vi "The Plant and its parameters (v. 2021).vi"() -> ()   [LabVIEW 2021]
uses:
  <vilib>/addons/control/pid/pid.llb/PID Advanced (DBL).vi
  <vilib>/addons/control/pid/NI_PID_pid.lvlib
panel:
  out "Chart 2":dbl(graph)
  out "u-1":dbl
  out "u":dbl
  out "tank level":dbl
  out "Plant Output":dbl(slide) scale=0.0..100.0
  out "Error test":bool
  out "value":bool
  out "control signal variation":T1(graph)
  out "?":dbl[][](array[numeric])
  in  "set point":dbl=85.0
  in  "PID parameter":cluster{"K":dbl, "Ti (min)":dbl, "Td (min)":dbl}={"K"=5.0, "Ti (min)"=0.005, "Td (min)"=0.0}
  in  "Plant Parameters":T2={"Static Gain"=1.0, "lag (s)"=5.0, "deadtime (s)"=0.2, "load"=20.0, "deadband"=0.0, "sensor noise"=0.0, "initial PV"=0.0, "plant noise"=10.0}
  in  "?":bool
  # "output value"
  # "time"
  # "error"
  # "Leakage"
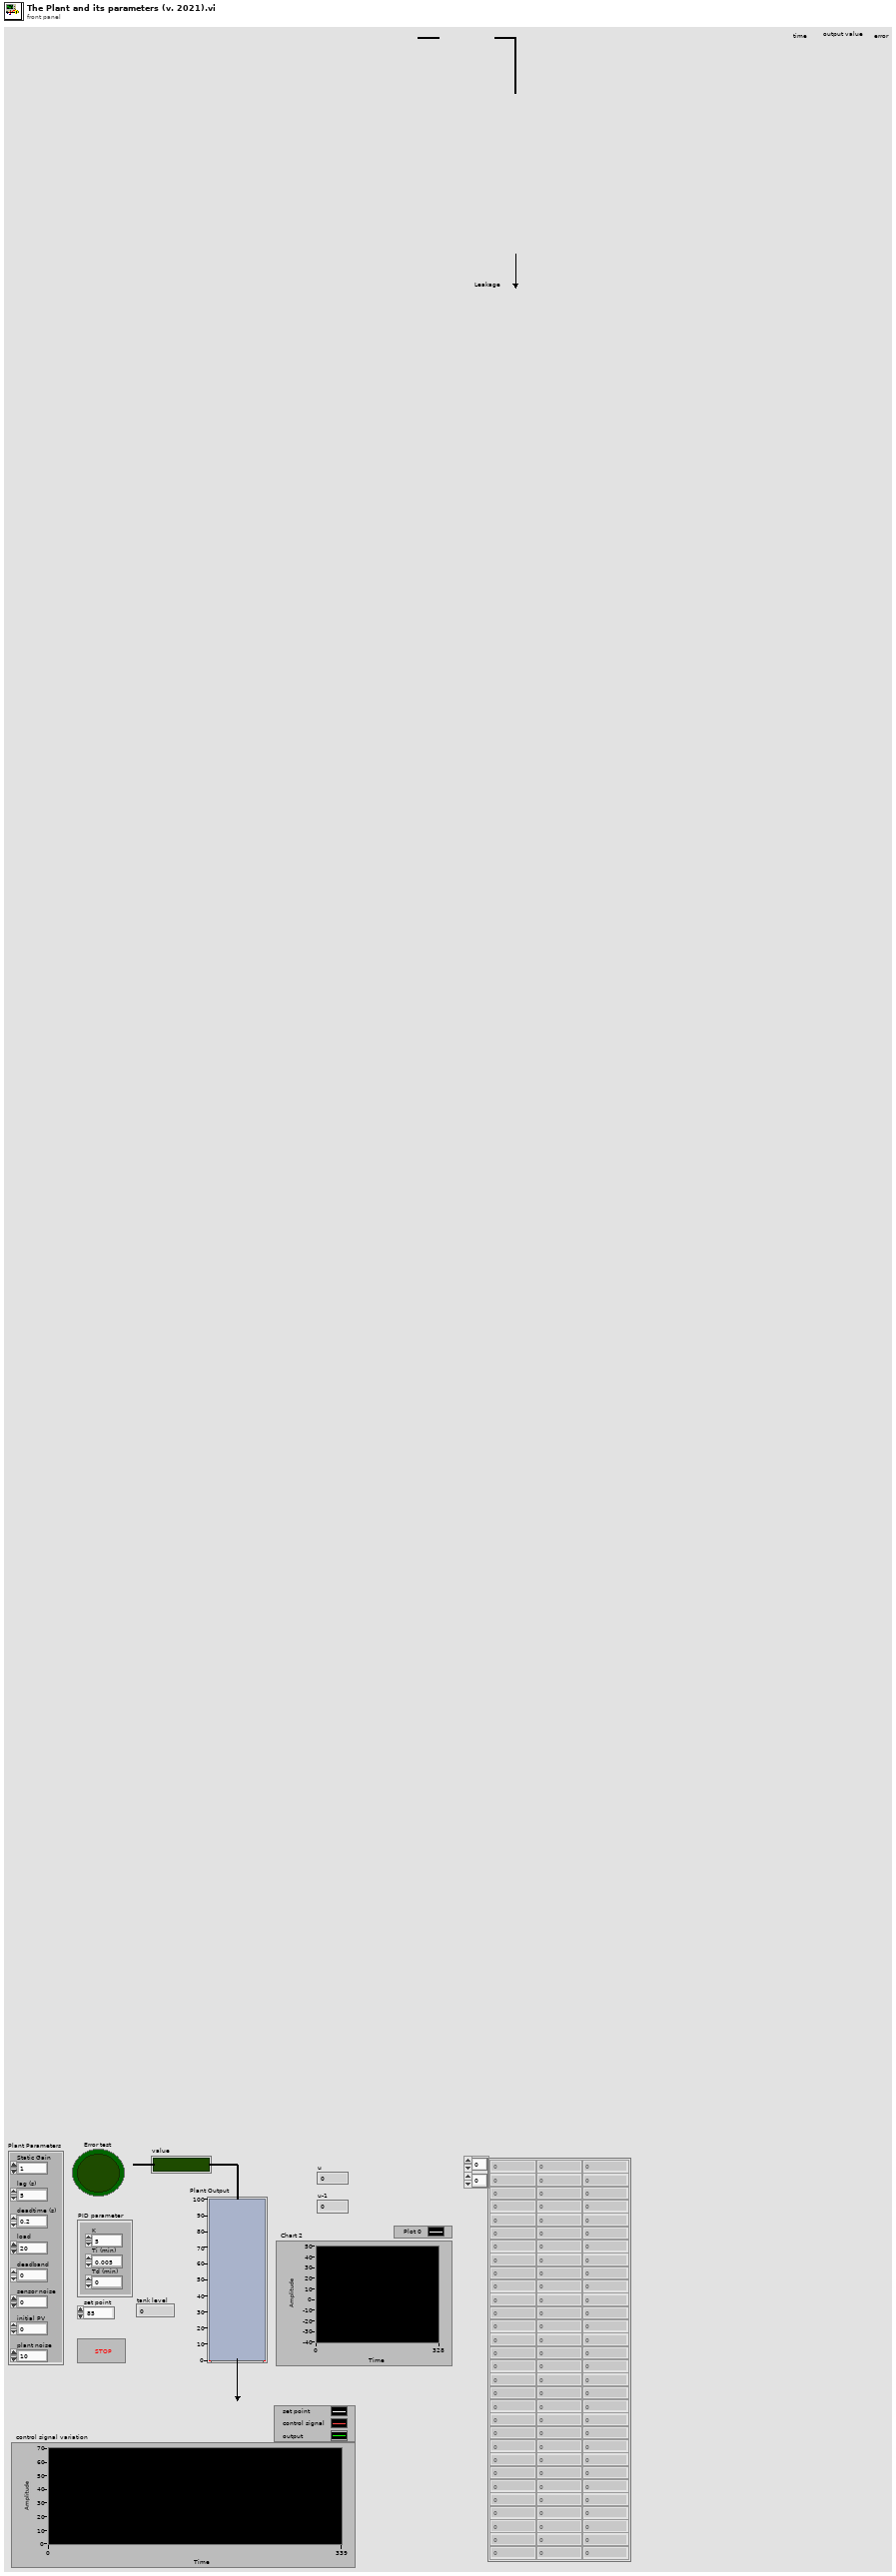
[diagram p1: front panel]
types:
  T1 = cluster{"set point":dbl, "output":dbl, "Plant Output":dbl}
  T2 = cluster{"Static Gain":dbl, "lag (s)":dbl, "deadtime (s)":dbl, "load":dbl, "deadband":dbl, "sensor noise":dbl, "initial PV":dbl, "plant noise":dbl}
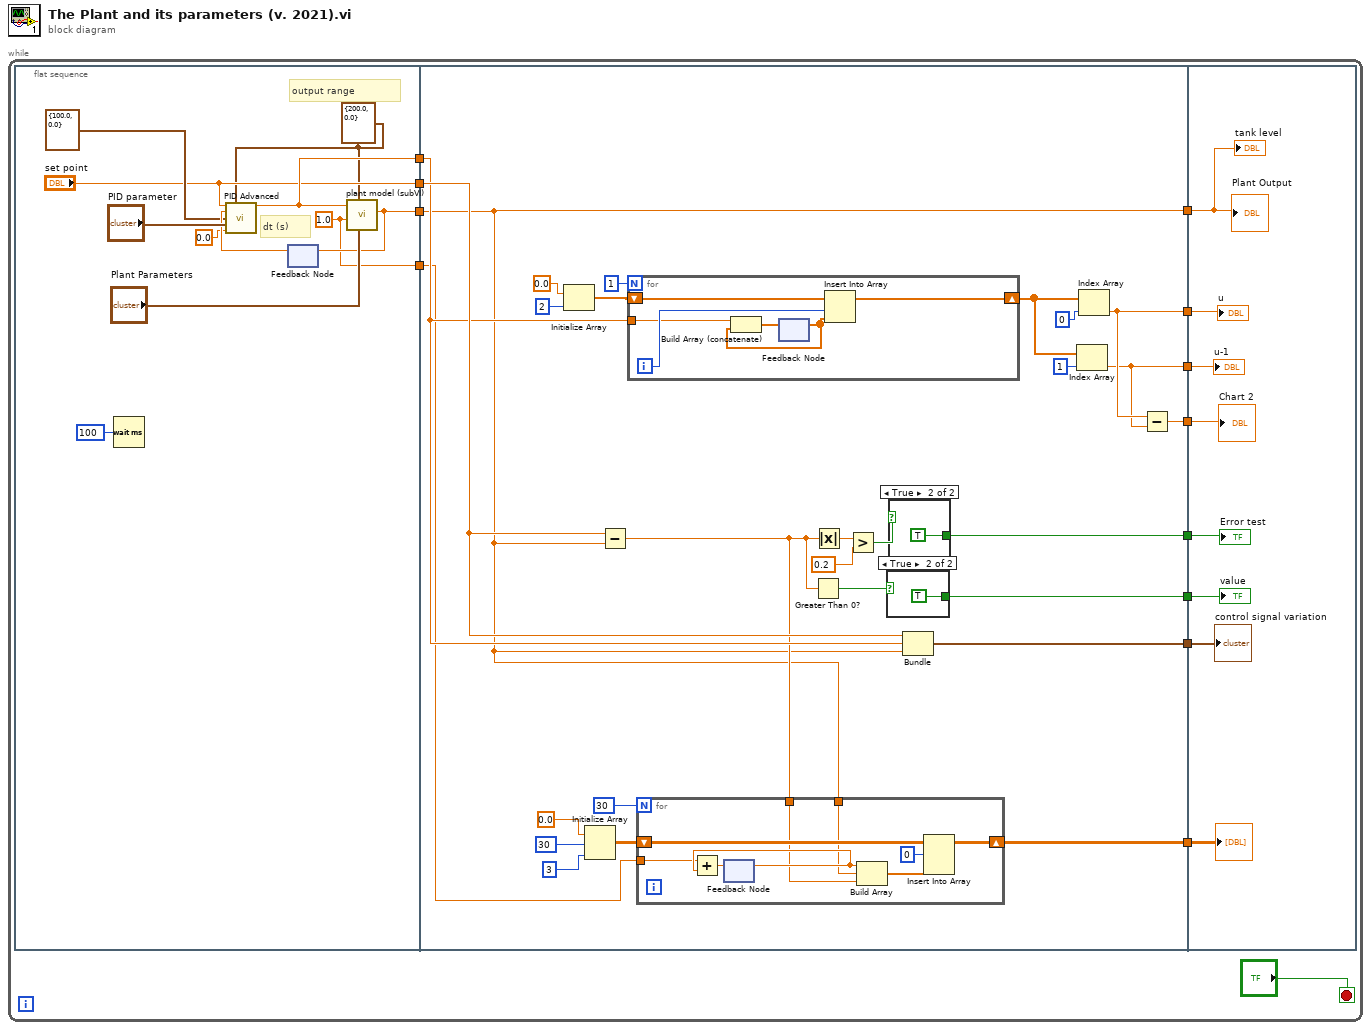
[diagram p0: block diagram]
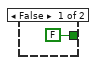
[diagram p2: hidden frame]
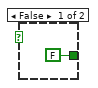
[diagram p3: hidden frame]
diagram:
  n1 = while {
    stop <- "?" stop-if-true
    n2 = flat-sequence {
      tunnel: [w19] -> w12
      tunnel: [w18] -> w11
      tunnel: ["set point"] -> w10
      tunnel: [w16] -> w1
      tunnel: w12 -> [w25]
      tunnel: w11 -> [w35]
      tunnel: w10 -> [w36]
      tunnel: [w34] -> w9
      tunnel: [w33] -> w8
      tunnel: [w32] -> w7
      tunnel: [w30] -> w6
      tunnel: [w29] -> w5
      tunnel: [w28] -> w4
      tunnel: [w27] -> w3
      tunnel: [w25] -> w2
      tunnel: w1 -> [w26]
      tunnel: w9 -> [w76]
      tunnel: w8 -> [w77]
      tunnel: w7 -> [w78]
      tunnel: w6 -> [w79]
      tunnel: w5 -> [w73]
      tunnel: w4 -> [w75]
      tunnel: w3 -> [w74]
      tunnel: w2 -> [w72]
      frame #0 {
        w14 = cluster{"output high":dbl, "output low":dbl} {"output high"=200.0, "output low"=0.0} ("output saturation range")
        w16 = 1.0 ("dt (s)")
        # "output range"
        # "dt (s)"
        n3 = Wait (ms)(milliseconds to wait=u32 100) -> ()  [unwired: 1 out]
        n4 = feedback #1() -> (w21:dbl)  [unwired: 1 in]
        n5 = call-poly <vilib>:"PID Advanced.vi"("setpoint"="set point", "output range"=w14, "process variable"=w21, "setpoint range"=cluster{"output high":dbl, "output low":dbl} {"output high"=100.0, "output low"=0.0} ("output saturation range"), "PID gains"="PID parameter", "dt (s)"=0.0) -> ("output"=w18:dbl)  [unwired: 8 in, 1 out]
        n6 = call "plant model (subVI).vi"("process parameters"="Plant Parameters", "output saturation range"=w14, "dt (s)"=w16, "Plant Input"=w18) -> ("Plant Output"=w19:dbl)  [unwired: 7 in]
        n7 = feedback-in #1(w19) -> ()
      }
      frame #1 {
        n8 = Initialize Array(0.0 ("element"), 2 ("dimension size")) -> (w37:dbl[])
        n9 = Initialize Array(0.0 ("element"), 30 ("dimension size"), 3 ("dimension size")) -> (w50:dbl[][])
        n10 = Subtract(x=w36, y=w25) -> (x-y=w31:dbl)
        n11 = for {
          N: 1 -> [_]
          shift-right: [w56] -> w41
          shift-left: w37 -> [w55]
          tunnel: w35 -> [w53]
          i -> [w54]
          n12 = feedback #2() -> (w57:dbl[])  [unwired: 1 in]
          n13 = Build Array (concatenate)(w53, w57) -> (w58:dbl[])
          n14 = feedback-in #2(w58) -> ()
          n15 = Insert Into Array(array=w55, index=w54, new element=w57) -> (w56:dbl[])
        }
        n16 = for {
          N: 30 -> [_]
          shift-right: [w69] -> w30
          shift-left: w50 -> [w68]
          tunnel: w25 -> [w65]
          tunnel: w31 -> [w64]
          tunnel: w26 -> [w63]
          n17 = feedback #3() -> (w66:dbl)  [unwired: 1 in]
          n18 = Add(x=w63, y=w66) -> (x+y=w67:dbl)
          n19 = feedback-in #3(w67) -> ()
          n20 = Build Array(w66, w65, w64) -> (w71:dbl[])
          n21 = Insert Into Array(array=w68, index (row)=0, new element=w71) -> (w69:dbl[][])  [unwired: 1 in]
        }
        n22 = Greater Than 0?(x=w31) -> (x > 0?=w44:bool)
        n23 = Absolute Value(x=w31) -> (abs(x)=w47:dbl)
        n24 = Greater?(x=w47, y=0.2) -> (0:w45:bool)
        n25 = case shown="True" w44 {
          tunnel: [FALSE ("value") TRUE ("value")] -> w33
          frame False {
          }
          frame True {
          }
        }
        n26 = case shown="True" w45 {
          tunnel: [FALSE ("Error test") TRUE ("Error test")] -> w34
          frame False {
          }
          frame True {
          }
        }
        n27 = Bundle("set point"=w36, "output"=w35, "Plant Output"=w25) -> (w32:T1)  [unwired: 1 in]
        n28 = Index Array(array=w41, index=1) -> (element=w27:dbl)
        n29 = Index Array(array=w41, index=0) -> (element=w28:dbl)
        n30 = Subtract(x=w28, y=w27) -> (x-y=w29:dbl)
      }
      frame #2 {
        "?" <- w79
        "control signal variation" <- w78
        "value" <- w77
        "Error test" <- w76
        "Plant Output" <- w72
        "tank level" <- w72
        "u" <- w75
        "u-1" <- w74
        "Chart 2" <- w73
      }
    }
  }
